vi "set AOI procedure.vi"(8 "error in (no error)":errorcluster, 11 "Thorcam in":refnum<class "Thorcam.lvclass">) -> (0 "error out":errorcluster, 3 "Thorcam out":refnum<class "Thorcam.lvclass">)   [LabVIEW 2012, in "Thorcam.lvclass"]
uses:
  Thorcam.lvclass
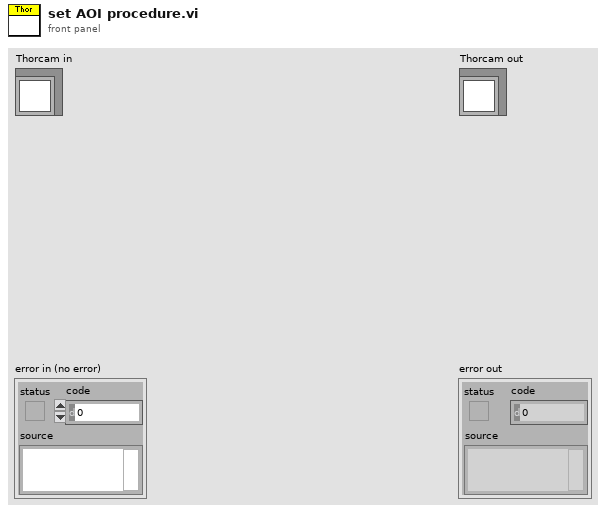
[diagram p1: front panel]
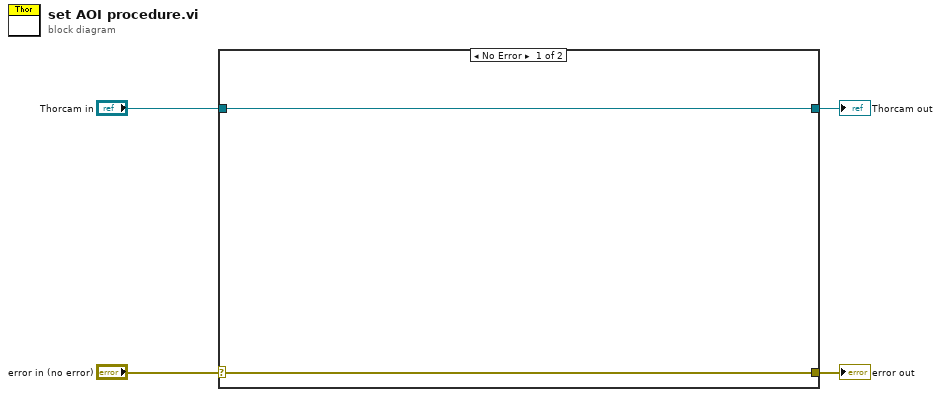
[diagram p0: block diagram]
diagram:
  n1 = case shown="No Error" "error in (no error)" {
    selector: "error in (no error)" -> [w5 w8]
    tunnel: [w5 w8] -> w3
    tunnel: [w6 w7] -> w1
    tunnel: "Thorcam in" -> [w6 w7]
    frame No Error {
    }
    frame Error {
    }
  }
  "error out" <- w3
  "Thorcam out" <- w1
